vi "Condition-Merge.vi"(8 "Any Start":dbl=10.0, 9 "Input Pos":cluster{"X":dbl, "Y":dbl, "Z":dbl}, 11 "All Lines":T1) -> (1 "Modified?":bool, 3 "array out":T1)   [LabVIEW 2014]
uses:
  Libraries/Map Data Folder/All-Lines.ctl
  Libraries/Map Data Folder/LineCluster.ctl
  Libraries/Map Data Folder/LineConnection.ctl
  Libraries/Map Data Folder/Map Data.lvlib
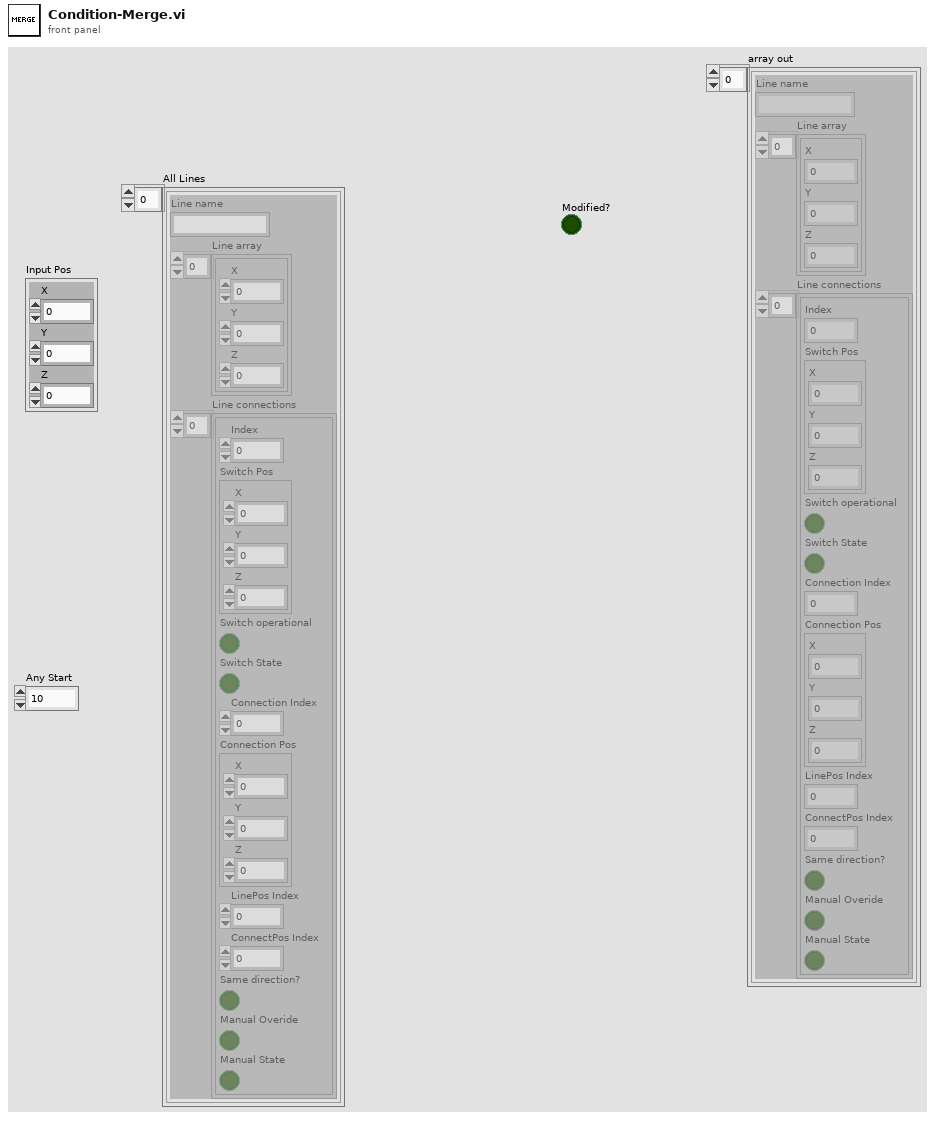
[diagram p1: front panel]
types:
  T1 = typedef "Map Data.lvlib/All-Lines.ctl" = T2[]
  T2 = typedef "Map Data.lvlib/LineCluster.ctl" = cluster{"Line name":string, "Line array":cluster{"X":dbl, "Y":dbl, "Z":dbl}[], "Line connections":T3[]}
  T3 = typedef "LineConnection.ctl" = cluster{"Index":i32, "Switch Pos":cluster{"X":dbl, "Y":dbl, "Z":dbl}, "Switch operational":bool, "Switch State":bool, "Connection Index":i32, "Connection Pos":cluster{"X":dbl, "Y":dbl, "Z":dbl}, "LinePos Index":i32, "ConnectPos Index":i32, "Same direction?":bool, "Manual Overide":bool, "Manual State":bool}
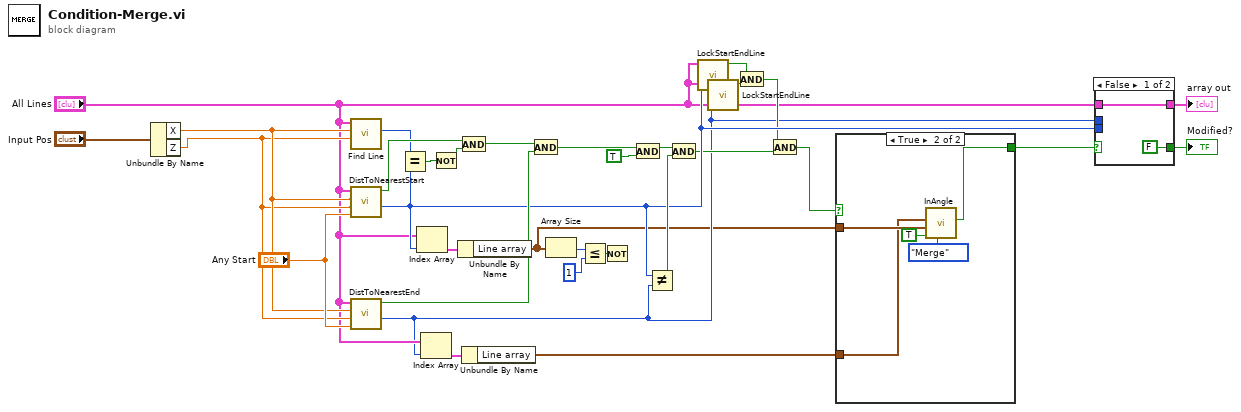
[diagram p0: block diagram]
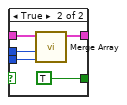
[diagram p3: hidden frame]
diagram:
  n1 = Unbundle By Name("Input Pos") -> ("X"=w17:dbl, "Z"=w16:dbl)
  n2 = call "Find Line.vi"("Z"=w16, "X"=w17, "All Lines"="All Lines") -> ("Nearest Line"=w15:i32)  [unwired: 5 in, 3 out]
  n3 = call "DistToNearestStart.vi"("Any Start"="Any Start", "Z"=w16, "X"=w17, "All Lines 2"="All Lines") -> ("Index"=w13:i32, "In range?"=w32:bool)  [unwired: 5 in, 1 out]
  n4 = call "DistToNearestEnd.vi"("Any End"="Any Start", "Z"=w16, "X"=w17, "All Lines 2"="All Lines") -> ("Index"=w6:i32, "In range?"=w26:bool)  [unwired: 5 in, 1 out]
  n5 = Equal?(x=w15, y=w13) -> (x = y?=w31:bool)
  n6 = Index Array(array="All Lines", index=w13) -> (element=w25:T2)
  n7 = Index Array(array="All Lines", index=w6) -> (element=w8:T2)
  n8 = Not(x=w31) -> (.not. x?=w29:bool)
  n9 = Unbundle By Name(w25) -> ("Line array"=w5:cluster{"X":dbl, "Y":dbl, "Z":dbl}[])
  n10 = And(x=w32, y=w29) -> (x .and. y?=w30:bool)
  n11 = Unbundle By Name(w8) -> ("Line array"=w4:cluster{"X":dbl, "Y":dbl, "Z":dbl}[])
  n12 = And(x=w30, y=w26) -> (x .and. y?=w28:bool)
  n13 = Array Size(array=w5) -> (size(s)=w24:i32)
  n14 = Less Or Equal?(x=w24, y=1) -> (x <= y?=w21:bool)
  n15 = Not(x=w21) -> ()  [unwired: 1 out]
  n16 = And(x=w28, y=TRUE) -> (x .and. y?=w22:bool)
  n17 = Not Equal?(x=w13, y=w6) -> (x != y?=w20:bool)
  n18 = And(x=w22, y=w20) -> (x .and. y?=w12:bool)
  n19 = call "LockStartEndLine.vi"("index"=w13, "All Lines"="All Lines") -> ("Not Locked?"=w11:bool)  [unwired: 9 in]
  n20 = call "LockStartEndLine.vi"("index"=w6, "All Lines"="All Lines") -> ("Not Locked?"=w10:bool)  [unwired: 9 in]
  n21 = And(x=w11, y=w10) -> (x .and. y?=w9:bool)
  n22 = And(x=w9, y=w12) -> (x .and. y?=w3:bool)
  n23 = case shown="True" w3 {
    selector: w3 -> [w33 _]
    tunnel: w5 -> [_ w38]
    tunnel: w4 -> [_ w37]
    tunnel: [w33 w36] -> w2
    frame False {
    }
    frame True {
      n24 = call "InAngle.vi"("Function"=enum16{"Posit", "Merge"}."Merge", "Towards Target?"=TRUE, "2nd Array (Start)"=w38, "Base Array (End)"=w37) -> ("In Angle?"=w36:bool)  [unwired: 7 in]
    }
  }
  n25 = case shown="False" w2 {
    tunnel: "All Lines" -> [w40 w45]
    tunnel: [w40 w44] -> w14
    tunnel: w13 -> [_ w43]
    tunnel: w6 -> [_ w42]
    tunnel: [FALSE ("y") TRUE ("y")] -> w1
    frame False {
    }
    frame True {
      n26 = call "Merge Array.vi"("Start array"=w43, "prev index"=w42, "array"=w45) -> ("array out"=w44:T1)  [unwired: 8 in]
    }
  }
  "array out" <- w14
  "Modified?" <- w1
